vi "Save VCSV.vi"(6 "Channel State":cluster{bool, bool, bool, bool}={TRUE, FALSE, FALSE, FALSE}, 8 "error in (no error)":errorcluster, 10 "TimeStamp":string="201711091600DSOS404", 11 "VISA resource name":refnum<visa-resource-name>="DSOS404") -> (0 "error out":errorcluster, 3 "VISA resource name out":refnum<visa-resource-name>="DSOS404")   [LabVIEW 2018]
panel:
  out "full file path":string
  # "CH1"
  # "CH2"
  # "CH3"
  # "CH4"
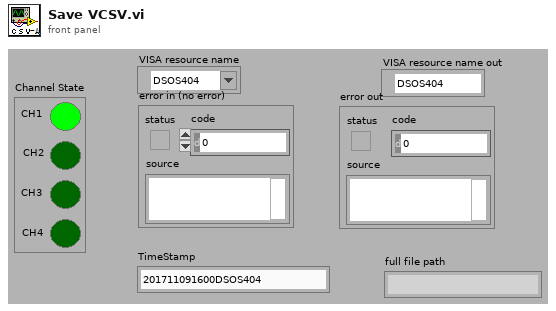
[diagram p1: front panel]
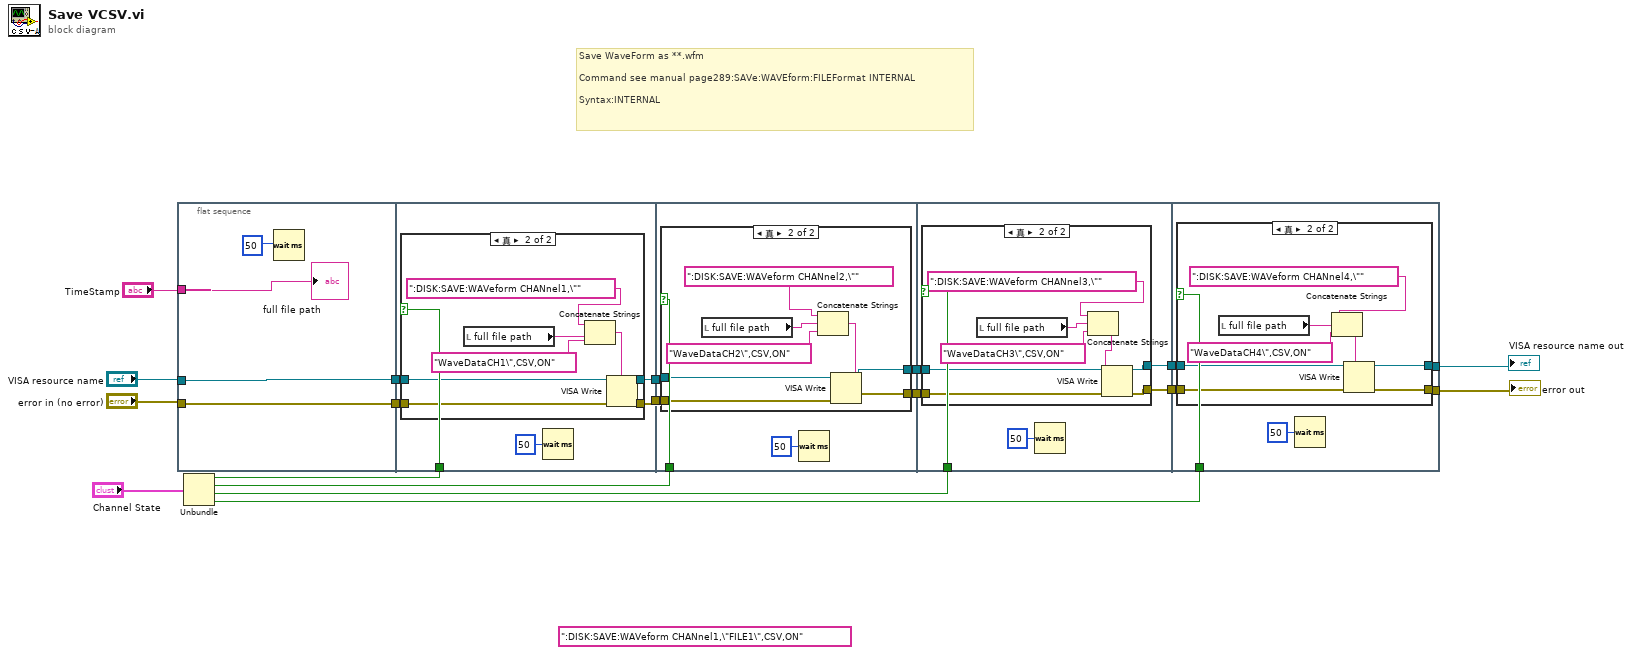
[diagram p0: block diagram]
diagram:
  (unwired) ":DISK:SAVE:WAVeform CHANnel1,\"FILE1\",CSV,ON" ("write buffer")
  # "Save WaveForm as **.wfm\n\nCommand see manual page289:SAVe:WAVEform:FILEFormat INTERNAL\n\nSyntax:INTERNAL"
  n1 = flat-sequence {
    tunnel: [w20] -> w18
    tunnel: [w19] -> w17
    tunnel: "TimeStamp" -> [w21]
    tunnel: "VISA resource name" -> [w20]
    tunnel: "error in (no error)" -> [w19]
    tunnel: [w28] -> w16
    tunnel: [w27] -> w15
    tunnel: w18 -> [w26]
    tunnel: w17 -> [w25]
    tunnel: w8 -> [w24]
    tunnel: w16 -> [w44]
    tunnel: w15 -> [w43]
    tunnel: [w42] -> w14
    tunnel: [w41] -> w13
    tunnel: w7 -> [w40]
    tunnel: w14 -> [w60]
    tunnel: w13 -> [w59]
    tunnel: [w58] -> w12
    tunnel: [w57] -> w11
    tunnel: w6 -> [w56]
    tunnel: [w74] -> w9
    tunnel: w12 -> [w76]
    tunnel: w11 -> [w75]
    tunnel: [w73] -> w4
    tunnel: w5 -> [w72]
    frame #0 {
      n2 = Wait (ms)(milliseconds to wait=u32 50) -> ()  [unwired: 1 out]
      "full file path" <- w21
    }
    frame #1 {
      n3 = case shown="真" w24 {
        tunnel: [w30 w38] -> w28
        tunnel: [w29 w37] -> w27
        tunnel: w26 -> [w30 w33]
        tunnel: w25 -> [w29 w32]
        frame False {
        }
        frame True {
          n4 = local read "full file path"() -> (w34:string)
          n5 = Concatenate Strings(":DISK:SAVE:WAVeform CHANnel1,\"" ("write buffer"), w34, "WaveDataCH1\",CSV,ON" ("format string")) -> (w35:string)
          n6 = VISA Write(VISA resource name=w33, write buffer=w35, error in (no error)=w32) -> (VISA resource name out=w38:refnum<visa-resource-name>, error out=w37:errorcluster)  [unwired: 1 out]
        }
      }
      n7 = Wait (ms)(milliseconds to wait=u32 50) -> ()  [unwired: 1 out]
    }
    frame #2 {
      n8 = case shown="真" w40 {
        tunnel: w44 -> [w46 w54]
        tunnel: w43 -> [w45 w53]
        tunnel: [w46 w52] -> w42
        tunnel: [w45 w51] -> w41
        frame False {
        }
        frame True {
          n9 = local read "full file path"() -> (w50:string)
          n10 = Concatenate Strings(":DISK:SAVE:WAVeform CHANnel2,\"" ("write buffer"), w50, "WaveDataCH2\",CSV,ON" ("format string")) -> (w48:string)
          n11 = VISA Write(VISA resource name=w54, write buffer=w48, error in (no error)=w53) -> (VISA resource name out=w52:refnum<visa-resource-name>, error out=w51:errorcluster)  [unwired: 1 out]
        }
      }
      n12 = Wait (ms)(milliseconds to wait=u32 50) -> ()  [unwired: 1 out]
    }
    frame #3 {
      n13 = case shown="真" w56 {
        tunnel: w60 -> [w62 w70]
        tunnel: w59 -> [w61 w69]
        tunnel: [w62 w68] -> w58
        tunnel: [w61 w67] -> w57
        frame False {
        }
        frame True {
          n14 = local read "full file path"() -> (w66:string)
          n15 = Concatenate Strings(":DISK:SAVE:WAVeform CHANnel3,\"" ("write buffer"), w66, "WaveDataCH3\",CSV,ON" ("format string")) -> (w64:string)
          n16 = VISA Write(VISA resource name=w70, write buffer=w64, error in (no error)=w69) -> (VISA resource name out=w68:refnum<visa-resource-name>, error out=w67:errorcluster)  [unwired: 1 out]
        }
      }
      n17 = Wait (ms)(milliseconds to wait=u32 50) -> ()  [unwired: 1 out]
    }
    frame #4 {
      n18 = case shown="真" w72 {
        tunnel: w76 -> [w78 w86]
        tunnel: w75 -> [w77 w85]
        tunnel: [w78 w82] -> w74
        tunnel: [w77 w81] -> w73
        frame False {
        }
        frame True {
          n19 = local read "full file path"() -> (w84:string)
          n20 = Concatenate Strings(":DISK:SAVE:WAVeform CHANnel4,\"" ("write buffer"), w84, "WaveDataCH4\",CSV,ON" ("format string")) -> (w80:string)
          n21 = VISA Write(VISA resource name=w86, write buffer=w80, error in (no error)=w85) -> (VISA resource name out=w82:refnum<visa-resource-name>, error out=w81:errorcluster)  [unwired: 1 out]
        }
      }
      n22 = Wait (ms)(milliseconds to wait=u32 50) -> ()  [unwired: 1 out]
    }
  }
  n23 = Unbundle("Channel State") -> (w8:bool, w7:bool, w6:bool, w5:bool)
  "VISA resource name out" <- w9
  "error out" <- w4
